vi "rsidr_core_global.vi"() -> ()   [LabVIEW 2020, in "Rohde&Schwarz CMWXP NR FR1 Measurement.lvlib"]
doc: "This Global variable contains driver's:\n- Attributes\n- Range Tables\n- Repeated Capabilities"
uses:
  <instrlib>/Rohde&Schwarz CMWXP NR FR1 Measurement/Rohde&Schwarz CMWXP NR FR1 Measurement.lvlib
panel:
  out "Attributes":T1(array[cluster])=[{"Level"=1, "Class Only"=TRUE, "Identifier"="", "Descriptive Name"="Configuration", "Data Type"=enum."ViInt32", "Command"="", "Access"=enum."Read Only", "Range Table"="", "Read Callback"="", "Write Callback"="", "Range Callback"="", "Check Callback"="", "Rngtable Callback"="", "Coerce Callback"="", "Supported Models"="", "Instrument Options"="", "Check Status Callback"="", "Flags"=0, "Help"="Contains attributes for configuring NR FR 1 Measurement."}, {"Level"=2, "Class Only"=FALSE, "Identifier"="RSCMWXPNRFR1M_ATTR_SIGNAL_PATH", "Descriptive Name"="Signal Path", "Data Type"=enum."RawString", "Command"="ROUT:NRS:MEAS{instance}:SCEN:SAL", "Access"=enum."Read/Write", "Range Table"="", "Read Callback"="", "Write Callback"="", "Range Callback"="", "Check Callback"="", "Rngtable Callback"="", "Coerce Callback"="", "Supported Models"="", "Instrument Options"="", "Check Status Callback"="", "Flags"=0, "Help"="Selects the signal path for the measured signal.\nValue combinations:\nRF 1 COM and RF 2 COM are compatible with TX 1 and TX 3.RF 3 COM and RF 4 COM are compatible with TX 2 and TX 4.\nNote: This command is an interim solution. It is planned to replace this command in a later software version.\n\nSyntax:\nROUTe:NRSub:MEAS<i>:SCENario:SALone <RXConnector>, <RFConverter>\n\n<RXConnector>\nRF connector for the input path\nSingle R&S CMW500: RF<n>C for RF <n> COM\nCMWflexx: R<a><b>C for CMW <a>, connector RF <b> COM\nValid Values:\nRF1C | RF2C | RF3C | RF4C | R11C | R12C | R13C | R14C | R21C | R22C | R23C | R24C | R31C | R32C | R33C | R34C | R41C | R42C | R43C | R44C\n\n<RFConverter>\nRX module for the input path\nSingle R&S CMW500: TX1 to TX4\nCMWflexx: TX<a><b> for CMW <a>, TX <b>\nValid Values:\nTX1 | TX2 | TX3 | TX4 | TX11 | TX12 | TX13 | TX14 | TX21 | TX22 | TX23 | TX24 | TX31 | TX32 | TX33 | TX34 | TX41 | TX42 | TX43 | TX44\n\nAvailable Repeated Capabilities:\ninstance: i0, i1, i2, i3, i4, i5, i6, i7, i8, i9, i10, i11, i12, i13, i14, i15, i16, i17, i18, i19, i20, i21, i22, i23, i24, i25, i26, i27, i28, i29, i30, i31, i32\r\n\nRemote-control command(s):\nROUTe:NRSub:MEAS<i>:SCENario:SALone"}, {"Level"=2, "Class Only"=FALSE, "Identifier"="RSCMWXPNRFR1M_ATTR_CONNECTOR", "Descriptive Name"="Connector", "Data Type"=enum."ViInt32", "Command"="CONF:NRS:MEAS{instance}:SPAT", "Access"=enum."Read/Write", "Range Table"="rsCmwxpNrFr1M_rngConnector", "Read Callback"="", "Write Callback"="", "Range Callback"="", "Check Callback"="", "Rngtable Callback"="", "Coerce Callback"="", "Supported Models"="", "Instrument Options"="", "Check Status Callback"="", "Flags"=0, "Help"="Selects between a standalone measurement and a measurement with coupling to signaling settings (cell settings of the network configuration).\n\nAvailable Repeated Capabilities:\ninstance: i0, i1, i2, i3, i4, i5, i6, i7, i8, i9, i10, i11, i12, i13, i14, i15, i16, i17, i18, i19, i20, i21, i22, i23, i24, i25, i26, i27, i28, i29, i30, i31, i32\r\n\nRemote-control command(s):\nCONFigure:NRSub:MEAS<i>:SPATh"}, {"Level"=2, "Class Only"=FALSE, "Identifier"="RSCMWXPNRFR1M_ATTR_EXTERNAL_ATTENUATION", "Descriptive Name"="External Attenuation", "Data Type"=enum."ViReal64", "Command"="CONF:NRS:MEAS{instance}:RFS:EATT", "Access"=enum."Read/Write", "Range Table"="rsCmwxpNrFr1M_rngExtAtt", "Read Callback"="", "Write Callback"="", "Range Callback"="", "Check Callback"="", "Rngtable Callback"="", "Coerce Callback"="", "Supported Models"="", "Instrument Options"="", "Check Status Callback"="", "Flags"=0, "Help"="Defines an external attenuation (or gain, if the value is negative), to be applied to the input connector.\n\nAvailable Repeated Capabilities:\ninstance: i0, i1, i2, i3, i4, i5, i6, i7, i8, i9, i10, i11, i12, i13, i14, i15, i16, i17, i18, i19, i20, i21, i22, i23, i24, i25, i26, i27, i28, i29, i30, i31, i32\r\n\nRemote-control command(s):\nCONFigure:NRSub:MEAS<i>:RFSettings:EATTenuation"}, {"Level"=2, "Class Only"=FALSE, "Identifier"="RSCMWXPNRFR1M_ATTR_BAND", "Descriptive Name"="Band", "Data Type"=enum."ViInt32", "Command"="CONF:NRS:MEAS{instance}:BAND", "Access"=enum."Read/Write", "Range Table"="rsCmwxpNrFr1M_rngBand", "Read Callback"="rscmwxpnrfr1m_OperatingBand_ReadCallback.vi", "Write Callback"="rscmwxpnrfr1m_OperatingBand_WriteCallback.vi", "Range Callback"="", "Check Callback"="", "Rngtable Callback"="", "Coerce Callback"="", "Supported Models"="", "Instrument Options"="", "Check Status Callback"="", "Flags"=0, "Help"="Selects the operating band (OB). The allowed input range depends on the duplex mode (FDD or TDD).\n\nAvailable Repeated Capabilities:\ninstance: i0, i1, i2, i3, i4, i5, i6, i7, i8, i9, i10, i11, i12, i13, i14, i15, i16, i17, i18, i19, i20, i21, i22, i23, i24, i25, i26, i27, i28, i29, i30, i31, i32\r\n\nRemote-control command(s):\nCONFigure:NRSub:MEAS<i>:BAND"}, {"Level"=2, "Class Only"=FALSE, "Identifier"="RSCMWXPNRFR1M_ATTR_FREQUENCY", "Descriptive Name"="Frequency", "Data Type"=enum."ViReal64", "Command"="CONF:NRS:MEAS{instance}:RFS:FREQ", "Access"=enum."Read/Write", "Range Table"="", "Read Callback"="", "Write Callback"="", "Range Callback"="", "Check Callback"="", "Rngtable Callback"="", "Coerce Callback"="", "Supported Models"="", "Instrument Options"="", "Check Status Callback"="", "Flags"=0, "Help"="Selects the center frequency of the measured carrier.\n\nAvailable Repeated Capabilities:\ninstance: i0, i1, i2, i3, i4, i5, i6, i7, i8, i9, i10, i11, i12, i13, i14, i15, i16, i17, i18, i19, i20, i21, i22, i23, i24, i25, i26, i27, i28, i29, i30, i31, i32\r\n\nRemote-control command(s):\nCONFigure:NRSub:MEAS<i>:RFSettings:FREQuency"}, {"Level"=2, "Class Only"=FALSE, "Identifier"="RSCMWXPNRFR1M_ATTR_FREQUENCY_OFFSET", "Descriptive Name"="Frequency Offset", "Data Type"=enum."ViReal64", "Command"="CONF:NRS:MEAS{instance}:RFS:FOFF", "Access"=enum."Read/Write", "Range Table"="rsCmwxpNrFr1M_rngFrequencyOffset", "Read Callback"="", "Write Callback"="", "Range Callback"="", "Check Callback"="", "Rngtable Callback"="", "Coerce Callback"="", "Supported Models"="", "Instrument Options"="", "Check Status Callback"="", "Flags"=0, "Help"="Specifies a positive or negative frequency offset to be added to the carrier center frequency.\n\nAvailable Repeated Capabilities:\ninstance: i0, i1, i2, i3, i4, i5, i6, i7, i8, i9, i10, i11, i12, i13, i14, i15, i16, i17, i18, i19, i20, i21, i22, i23, i24, i25, i26, i27, i28, i29, i30, i31, i32\r\n\nRemote-control command(s):\nCONFigure:NRSub:MEAS<i>:RFSettings:FOFFset"}, {"Level"=2, "Class Only"=FALSE, "Identifier"="RSCMWXPNRFR1M_ATTR_EXPECTED_NOMINAL_POWER", "Descriptive Name"="Expected Nominal Power", "Data Type"=enum."ViReal64", "Command"="CONF:NRS:MEAS{instance}:RFS:ENP", "Access"=enum."Read/Write", "Range Table"="", "Read Callback"="", "Write Callback"="", "Range Callback"="", "Check Callback"="", "Rngtable Callback"="", "Coerce Callback"="", "Supported Models"="", "Instrument Options"="", "Check Status Callback"="", "Flags"=0, "Help"="Sets the expected nominal power of the measured RF signal.\n\nAvailable Repeated Capabilities:\ninstance: i0, i1, i2, i3, i4, i5, i6, i7, i8, i9, i10, i11, i12, i13, i14, i15, i16, i17, i18, i19, i20, i21, i22, i23, i24, i25, i26, i27, i28, i29, i30, i31, i32\r\n\nRemote-control command(s):\nCONFigure:NRSub:MEAS<i>:RFSettings:ENPower"}, {"Level"=2, "Class Only"=FALSE, "Identifier"="RSCMWXPNRFR1M_ATTR_USER_MARGIN", "Descriptive Name"="User Margin", "Data Type"=enum."ViReal64", "Command"="CONF:NRS:MEAS{instance}:RFS:UMAR", "Access"=enum."Read/Write", "Range Table"="", "Read Callback"="", "Write Callback"="", "Range Callback"="", "Check Callback"="", "Rngtable Callback"="", "Coerce Callback"="", "Supported Models"="", "Instrument Options"="", "Check Status Callback"="", "Flags"=0, "Help"="Sets the margin that the measurement adds to the expected nominal power to determine the reference power. The reference power minus the external input attenuation must be within the power range of the selected input connector. Refer to the data sheet.\n\nAvailable Repeated Capabilities:\ninstance: i0, i1, i2, i3, i4, i5, i6, i7, i8, i9, i10, i11, i12, i13, i14, i15, i16, i17, i18, i19, i20, i21, i22, i23, i24, i25, i26, i27, i28, i29, i30, i31, i32\r\n\nRemote-control command(s):\nCONFigure:NRSub:MEAS<i>:RFSettings:UMARgin"}, {"Level"=2, "Class Only"=FALSE, "Identifier"="RSCMWXPNRFR1M_ATTR_MIXER_LEVEL_OFFSET", "Descriptive Name"="Mixer Level Offset", "Data Type"=enum."ViReal64", "Command"="CONF:NRS:MEAS{instance}:RFS:MLOF", "Access"=enum."Read/Write", "Range Table"="rsCmwxpNrFr1M_rngMixerLevelOffset", "Read Callback"="", "Write Callback"="", "Range Callback"="", "Check Callback"="", "Rngtable Callback"="", "Coerce Callback"="", "Supported Models"="", "Instrument Options"="", "Check Status Callback"="", "Flags"=0, "Help"="Varies the input level of the mixer in the analyzer path.\n\nAvailable Repeated Capabilities:\ninstance: i0, i1, i2, i3, i4, i5, i6, i7, i8, i9, i10, i11, i12, i13, i14, i15, i16, i17, i18, i19, i20, i21, i22, i23, i24, i25, i26, i27, i28, i29, i30, i31, i32\r\n\nRemote-control command(s):\nCONFigure:NRSub:MEAS<i>:RFSettings:MLOFfset"}, {"Level"=2, "Class Only"=FALSE, "Identifier"="RSCMWXPNRFR1M_ATTR_RF_UPCONVERSION", "Descriptive Name"="RF Upconversion", "Data Type"=enum."RawString", "Command"="CONF:NRS:MEAS{instance}:MEV:PCOM", "Access"=enum."Read/Write", "Range Table"="", "Read Callback"="", "Write Callback"="", "Range Callback"="", "Check Callback"="", "Rngtable Callback"="", "Coerce Callback"="", "Supported Models"="", "Instrument Options"="", "Check Status Callback"="", "Flags"=0, "Help"="Specifies the phase compensation applied by the UE during the modulation and upconversion.\n\nSyntax:\nCONFigure:NRSub:MEAS<i>:MEValuation:PCOMp <PhaseComp>, <UserDefFreq>\n\n<PhaseComp>\nValid Values:\nOFF: no phase compensation\nCAF: phase compensation for carrier frequency\nUDEF: phase compensation for frequency <UserDefFreq>\n \n<UserDefFreq>\n numeric\nFrequency for <PhaseComp> = UDEF\nValid Values: 0 Hz to 10E+9 Hz\n\nAvailable Repeated Capabilities:\ninstance: i0, i1, i2, i3, i4, i5, i6, i7, i8, i9, i10, i11, i12, i13, i14, i15, i16, i17, i18, i19, i20, i21, i22, i23, i24, i25, i26, i27, i28, i29, i30, i31, i32\r\n\nRemote-control command(s):\nCONFigure:NRSub:MEAS<i>:MEValuation:PCOMp"}, {"Level"=2, "Class Only"=FALSE, "Identifier"="RSCMWXPNRFR1M_ATTR_DUPLEX_MODE", "Descriptive Name"="Duplex Mode", "Data Type"=enum."ViInt32", "Command"="CONF:NRS:MEAS{instance}:MEV:DMOD", "Access"=enum."Read/Write", "Range Table"="rsCmwxpNrFr1M_rngDuplexMode", "Read Callback"="", "Write Callback"="", "Range Callback"="", "Check Callback"="", "Rngtable Callback"="", "Coerce Callback"="", "Supported Models"="", "Instrument Options"="", "Check Status Callback"="", "Flags"=0, "Help"="Selects the duplex mode of the signal: FDD or TDD.\n\nAvailable Repeated Capabilities:\ninstance: i0, i1, i2, i3, i4, i5, i6, i7, i8, i9, i10, i11, i12, i13, i14, i15, i16, i17, i18, i19, i20, i21, i22, i23, i24, i25, i26, i27, i28, i29, i30, i31, i32\r\n\nRemote-control command(s):\nCONFigure:NRSub:MEAS<i>:MEValuation:DMODe"}, {"Level"=2, "Class Only"=FALSE, "Identifier"="RSCMWXPNRFR1M_ATTR_EN_DC_MODE", "Descriptive Name"="EN-DC Mode", "Data Type"=enum."ViBoolean", "Command"="CONF:NRS:MEAS{instance}:MEV:ENDC", "Access"=enum."Read/Write", "Range Table"="", "Read Callback"="", "Write Callback"="", "Range Callback"="", "Check Callback"="", "Rngtable Callback"="", "Coerce Callback"="", "Supported Models"="", "Instrument Options"="", "Check Status Callback"="", "Flags"=0, "Help"="Enables or disables the EN-DC mode of the measurement.\n\nAvailable Repeated Capabilities:\ninstance: i0, i1, i2, i3, i4, i5, i6, i7, i8, i9, i10, i11, i12, i13, i14, i15, i16, i17, i18, i19, i20, i21, i22, i23, i24, i25, i26, i27, i28, i29, i30, i31, i32\r\n\nRemote-control command(s):\nCONFigure:NRSub:MEAS<i>:MEValuation:ENDC"}, {"Level"=2, "Class Only"=FALSE, "Identifier"="RSCMWXPNRFR1M_ATTR_EN_DC_LTE", "Descriptive Name"="EN-DC LTE", "Data Type"=enum."RawString", "Command"="CONF:NRS:MEAS{instance}:MEV:ENDC:EUTR", "Access"=enum."Read/Write", "Range Table"="", "Read Callback"="", "Write Callback"="", "Range Callback"="", "Check Callback"="", "Rngtable Callback"="", "Coerce Callback"="", "Supported Models"="", "Instrument Options"="", "Check Status Callback"="", "Flags"=0, "Help"="Configures LTE settings for EN-DC.\n\nSyntax:\nCONFigure:NRSub:MEAS<i>:MEValuation:ENDC:EUTRa <ChannelBW>, <CarrierPosition>\n\n<ChannelBW>\nChannel bandwidth in MHz (5 MHz to 20 MHz)\nValid Values:\nB005 | B010 | B015 | B020\n\n<CarrierPosition>\nPosition of LTE carrier left (LONR) or right (RONR) of NR carrier.\nValid Values:\nLONR | RONR\n\nAvailable Repeated Capabilities:\ninstance: i0, i1, i2, i3, i4, i5, i6, i7, i8, i9, i10, i11, i12, i13, i14, i15, i16, i17, i18, i19, i20, i21, i22, i23, i24, i25, i26, i27, i28, i29, i30, i31, i32\r\n\nRemote-control command(s):\nCONFigure:NRSub:MEAS<i>:MEValuation:ENDC:EUTRa"}, {"Level"=2, "Class Only"=FALSE, "Identifier"="RSCMWXPNRFR1M_ATTR_TX_BANDWIDTH_OFFSET", "Descriptive Name"="Tx Bandwidth Offset", "Data Type"=enum."ViInt32", "Command"="CONF:NRS:MEAS{instance}:CC{CC}:TXBW:OFFS", "Access"=enum."Read/Write", "Range Table"="rsCmwxpNrFr1M_rngTxBWOffset", "Read Callback"="", "Write Callback"="", "Range Callback"="", "Check Callback"="", "Rngtable Callback"="", "Coerce Callback"="", "Supported Models"="", "Instrument Options"="", "Check Status Callback"="", "Flags"=0, "Help"="Specifies the offset to carrier (TxBW offset) of carrier <no>.\n\nAvailable Repeated Capabilities:\ninstance: i0, i1, i2, i3, i4, i5, i6, i7, i8, i9, i10, i11, i12, i13, i14, i15, i16, i17, i18, i19, i20, i21, i22, i23, i24, i25, i26, i27, i28, i29, i30, i31, i32\r\nCC: cc1, cc2\r\n\nRemote-control command(s):\nCONFigure:NRSub:MEAS<i>[:CC<no>]:TXBWidth:OFFSet"}, {"Level"=2, "Class Only"=TRUE, "Identifier"="", "Descriptive Name"="Signal Settings", "Data Type"=enum."ViInt32", "Command"="", "Access"=enum."Read Only", "Range Table"="", "Read Callback"="", "Write Callback"="", "Range Callback"="", "Check Callback"="", "Rngtable Callback"="", "Coerce Callback"="", "Supported Models"="", "Instrument Options"="", "Check Status Callback"="", "Flags"=0, "Help"="Describe properties of the measured NR signal, that are needed for synchronization and decoding."}, {"Level"=3, "Class Only"=TRUE, "Identifier"="", "Descriptive Name"="TDD UL-DL Configuration", "Data Type"=enum."ViInt32", "Command"="", "Access"=enum."Read Only", "Range Table"="", "Read Callback"="", "Write Callback"="", "Range Callback"="", "Check Callback"="", "Rngtable Callback"="", "Coerce Callback"="", "Supported Models"="", "Instrument Options"="", "Check Status Callback"="", "Flags"=0, "Help"="Settings that configure the UL-DL pattern."}, {"Level"=4, "Class Only"=FALSE, "Identifier"="RSCMWXPNRFR1M_ATTR_UL_DL_PERIODICITY", "Descriptive Name"="UL-DL Periodicity", "Data Type"=enum."ViInt32", "Command"="CONF:NRS:MEAS{instance}:ULDL:PER", "Access"=enum."Read/Write", "Range Table"="rsCmwxpNrFr1M_rngPeriodicity", "Read Callback"="", "Write Callback"="", "Range Callback"="", "Check Callback"="", "Rngtable Callback"="", "Coerce Callback"="", "Supported Models"="", "Instrument Options"="", "Check Status Callback"="", "Flags"=0, "Help"="Configures the periodicity of the TDD UL-DL pattern.\n\nAvailable Repeated Capabilities:\ninstance: i0, i1, i2, i3, i4, i5, i6, i7, i8, i9, i10, i11, i12, i13, i14, i15, i16, i17, i18, i19, i20, i21, i22, i23, i24, i25, i26, i27, i28, i29, i30, i31, i32\r\n\nRemote-control command(s):\nCONFigure:NRSub:MEAS<i>:ULDL:PERiodicity"}, {"Level"=4, "Class Only"=FALSE, "Identifier"="RSCMWXPNRFR1M_ATTR_UL_DL_PATTERN", "Descriptive Name"="UL-DL Pattern", "Data Type"=enum."RawString", "Command"="CONF:NRS:MEAS{instance}:ULDL:PATT", "Access"=enum."Write Only", "Range Table"="", "Read Callback"="", "Write Callback"="", "Range Callback"="", "Check Callback"="", "Rngtable Callback"="", "Coerce Callback"="", "Supported Models"="", "Instrument Options"="", "Check Status Callback"="", "Flags"=0, "Help"="Configures the UL-DL pattern for the <SCSpacing>.\n\nSyntax:\nCONFigure:NRMMw:MEAS<i>:ULDL:PATTern <SCSpacing>, <DLSlots>, <DLSymbols>, <ULSlots>, <ULSymbols>\n\n<SCSpacing>\nSubcarrier spacing for which the other settings apply.\nValid Values:\nS60K\nS120k\n\n<DLSlots>\nnumeric\nSpecifies nrofDownlinkSlots.\nValid Values:  0  to  78 \n\n<DLSymbols>\n numeric\nSpecifies nrofDownlinkSymbols.\nValid Values: 0 to 14 \n\n<ULSlots>\n numeric\nSpecifies nrofUplinkSlots.\nValid Values: 1 to 80 \n\n<ULSymbols>\nnumeric\nSpecifies nrofUplinkSymbols.\nValid Values: 0 to 14\n\nAvailable Repeated Capabilities:\ninstance: i0, i1, i2, i3, i4, i5, i6, i7, i8, i9, i10, i11, i12, i13, i14, i15, i16, i17, i18, i19, i20, i21, i22, i23, i24, i25, i26, i27, i28, i29, i30, i31, i32\r\n\nRemote-control command(s):\nCONFigure:NRSub:MEAS<i>:ULDL:PATTern"}, {"Level"=4, "Class Only"=FALSE, "Identifier"="RSCMWXPNRFR1M_ATTR_HIDDEN_QUERY_UL_DL_PATTERN", "Descriptive Name"="Query UL-DL Pattern", "Data Type"=enum."RawString", "Command"="CONF:NRS:MEAS{instance}:ULDL:PATT?", "Access"=enum."Read Only", "Range Table"="", "Read Callback"="", "Write Callback"="", "Range Callback"="", "Check Callback"="", "Rngtable Callback"="", "Coerce Callback"="", "Supported Models"="", "Instrument Options"="", "Check Status Callback"="", "Flags"=8, "Help"="Retrives the UL-DL pattern for the <SCSpacing>.\n\nSyntax:\nCONFigure:NRMMw:MEAS<i>:ULDL:PATTern? <SCSpacing>\n\nParameters:\n<SCSpacing>\nSubcarrier spacing for which the other settings apply.\nValid Values:\nS60K\nS120k\n\nResponse:\n<DLSlots>\nnumeric\nSpecifies nrofDownlinkSlots.\nValid Values:  0  to  78 \n\n<DLSymbols>\n numeric\nSpecifies nrofDownlinkSymbols.\nValid Values: 0 to 14 \n\n<ULSlots>\n numeric\nSpecifies nrofUplinkSlots.\nValid Values: 1 to 80 \n\n<ULSymbols>\nnumeric\nSpecifies nrofUplinkSymbols.\nValid Values: 0 to 14\n\nAvailable Repeated Capabilities:\ninstance: i0, i1, i2, i3, i4, i5, i6, i7, i8, i9, i10, i11, i12, i13, i14, i15, i16, i17, i18, i19, i20, i21, i22, i23, i24, i25, i26, i27, i28, i29, i30, i31, i32\r\n\nRemote-control command(s):\nCONFigure:NRSub:MEAS<i>:ULDL:PATTern?"}, {"Level"=3, "Class Only"=TRUE, "Identifier"="", "Descriptive Name"="General Carrier Settings", "Data Type"=enum."ViInt32", "Command"="", "Access"=enum."Read Only", "Range Table"="", "Read Callback"="", "Write Callback"="", "Range Callback"="", "Check Callback"="", "Rngtable Callback"="", "Coerce Callback"="", "Supported Models"="", "Instrument Options"="", "Check Status Callback"="", "Flags"=0, "Help"="General carrier settings."}, {"Level"=4, "Class Only"=FALSE, "Identifier"="RSCMWXPNRFR1M_ATTR_CHANNEL_BANDWIDTH", "Descriptive Name"="Channel Bandwidth", "Data Type"=enum."ViInt32", "Command"="CONF:NRS:MEAS{instance}:CC{CC}:CBAN", "Access"=enum."Read/Write", "Range Table"="rsCmwxpNrFr1M_rngChannelBandwidth", "Read Callback"="", "Write Callback"="", "Range Callback"="", "Check Callback"="", "Rngtable Callback"="", "Coerce Callback"="", "Supported Models"="", "Instrument Options"="", "Check Status Callback"="", "Flags"=0, "Help"="Specifies the channel bandwidth of carrier <no>.\n\nAvailable Repeated Capabilities:\ninstance: i0, i1, i2, i3, i4, i5, i6, i7, i8, i9, i10, i11, i12, i13, i14, i15, i16, i17, i18, i19, i20, i21, i22, i23, i24, i25, i26, i27, i28, i29, i30, i31, i32\r\nCC: cc1, cc2\r\n\nRemote-control command(s):\nCONFigure:NRSub:MEAS<i>[:CC<no>]:CBANdwidth"}, {"Level"=4, "Class Only"=FALSE, "Identifier"="RSCMWXPNRFR1M_ATTR_PHYSICAL_CELL_ID", "Descriptive Name"="Physical Cell ID", "Data Type"=enum."ViInt32", "Command"="CONF:NRS:MEAS{instance}:CC{CC}:PLC", "Access"=enum."Read/Write", "Range Table"="rsCmwxpNrFr1M_rngPhysicalCellID", "Read Callback"="", "Write Callback"="", "Range Callback"="", "Check Callback"="", "Rngtable Callback"="", "Coerce Callback"="", "Supported Models"="", "Instrument Options"="", "Check Status Callback"="", "Flags"=0, "Help"="Specifies the physical cell ID of carrier <no>.\n\nAvailable Repeated Capabilities:\ninstance: i0, i1, i2, i3, i4, i5, i6, i7, i8, i9, i10, i11, i12, i13, i14, i15, i16, i17, i18, i19, i20, i21, i22, i23, i24, i25, i26, i27, i28, i29, i30, i31, i32\r\nCC: cc1, cc2\r\n\nRemote-control command(s):\nCONFigure:NRSub:MEAS<i>[:CC<no>]:PLCid"}, {"Level"=4, "Class Only"=FALSE, "Identifier"="RSCMWXPNRFR1M_ATTR_DMRS_TYPE_A_POSITION", "Descriptive Name"="DMRS Type A Position", "Data Type"=enum."ViInt32", "Command"="CONF:NRS:MEAS{instance}:CC{CC}:TAP", "Access"=enum."Read/Write", "Range Table"="rsCmwxpNrFr1M_rngTypeAPosition", "Read Callback"="", "Write Callback"="", "Range Callback"="", "Check Callback"="", "Rngtable Callback"="", "Coerce Callback"="", "Supported Models"="", "Instrument Options"="", "Check Status Callback"="", "Flags"=0, "Help"="Specifies the 'dmrs-TypeA-Position' for carrier <no>.\n\nAvailable Repeated Capabilities:\ninstance: i0, i1, i2, i3, i4, i5, i6, i7, i8, i9, i10, i11, i12, i13, i14, i15, i16, i17, i18, i19, i20, i21, i22, i23, i24, i25, i26, i27, i28, i29, i30, i31, i32\r\nCC: cc1, cc2\r\n\nRemote-control command(s):\nCONFigure:NRSub:MEAS<i>[:CC<no>]:TAPosition"}, {"Level"=4, "Class Only"=FALSE, "Identifier"="RSCMWXPNRFR1M_ATTR_SUBCARRIER_SPACING", "Descriptive Name"="Subcarrier Spacing", "Data Type"=enum."ViInt32", "Command"="CONF:NRS:MEAS{instance}:CCAL:TXBW:SCSP", "Access"=enum."Read/Write", "Range Table"="rsCmwxpNrFr1M_rngSubcarrierSpacing", "Read Callback"="", "Write Callback"="", "Range Callback"="", "Check Callback"="", "Rngtable Callback"="", "Coerce Callback"="", "Supported Models"="", "Instrument Options"="", "Check Status Callback"="", "Flags"=0, "Help"="Selects the subcarrier spacing for the measurement, for all carriers.\n\nAvailable Repeated Capabilities:\ninstance: i0, i1, i2, i3, i4, i5, i6, i7, i8, i9, i10, i11, i12, i13, i14, i15, i16, i17, i18, i19, i20, i21, i22, i23, i24, i25, i26, i27, i28, i29, i30, i31, i32\r\n\nRemote-control command(s):\nCONFigure:NRSub:MEAS<i>:CCALl:TXBWidth:SCSPacing"}, {"Level"=3, "Class Only"=TRUE, "Identifier"="", "Descriptive Name"="Bandwidth Parts", "Data Type"=enum."ViInt32", "Command"="", "Access"=enum."Read Only", "Range Table"="", "Read Callback"="", "Write Callback"="", "Range Callback"="", "Check Callback"="", "Rngtable Callback"="", "Coerce Callback"="", "Supported Models"="", "Instrument Options"="", "Check Status Callback"="", "Flags"=0, "Help"="Contains attributes for Bandwidth Parts."}, {"Level"=4, "Class Only"=FALSE, "Identifier"="RSCMWXPNRFR1M_ATTR_BANDWIDTH_PART", "Descriptive Name"="Bandwidth Part", "Data Type"=enum."RawString", "Command"="CONF:NRS:MEAS{instance}:CC{CC}:BWP", "Access"=enum."Write Only", "Range Table"="", "Read Callback"="", "Write Callback"="", "Range Callback"="", "Check Callback"="", "Rngtable Callback"="", "Coerce Callback"="", "Supported Models"="", "Instrument Options"="", "Check Status Callback"="", "Flags"=0, "Help"="Configures basic properties of the <BWP> on carrier <CC>.\n\nSyntax:\nCONFigure:NRSub:MEAS<i>[:CC<no>]:BWPart <BWP>, <SCSpacing>, <CyclicPrefix>, <NumberRB>, <StartRB>\n\n<BWP>\nSelects BWP.\nValid Values:\nBWP0\n\n<SCSpacing>\nSubcarrier spacing 15 kHz, 30 kHz, 60 kHz.\nValid Values:\nS15K\nS30K\nS60K\n\n<CyclicPrefix>\nOnly normal CP is supported.\nValid Values:\nNORM\nEXT\n\n<NumberRB>\nNumber of RBs in the bandwidth part.\ninteger\nValid Values: 11 to 273 \n\n<StartRB>\nIndex of the first RB in the bandwidth part.\ninteger\nValid Values: 0 to 262\n\nAvailable Repeated Capabilities:\ninstance: i0, i1, i2, i3, i4, i5, i6, i7, i8, i9, i10, i11, i12, i13, i14, i15, i16, i17, i18, i19, i20, i21, i22, i23, i24, i25, i26, i27, i28, i29, i30, i31, i32\r\nCC: cc1, cc2\r\n\nRemote-control command(s):\nCONFigure:NRSub:MEAS<i>[:CC<no>]:BWPart"}, {"Level"=4, "Class Only"=FALSE, "Identifier"="RSCMWXPNRFR1M_ATTR_HIDDEN_QUERY_BANDWIDTH_PART", "Descriptive Name"="Query Bandwidth Part", "Data Type"=enum."RawString", "Command"="CONF:NRS:MEAS{instance}:CC{CC}:BWP?", "Access"=enum."Read Only", "Range Table"="", "Read Callback"="", "Write Callback"="", "Range Callback"="", "Check Callback"="", "Rngtable Callback"="", "Coerce Callback"="", "Supported Models"="", "Instrument Options"="", "Check Status Callback"="", "Flags"=8, "Help"="Queries basic properties of the <BWP> on carrier <CC>.\n\nSyntax:\nCONFigure:NRSub:MEAS<i>[:CC<no>]:BWPart? <BWP>\n\nParameters:\n<BWP>\nSelects BWP.\nValid Values:\nBWP0\n\nResponse:\n<SCSpacing>\nSubcarrier spacing 15 kHz, 30 kHz, 60 kHz.\nValid Values:\nS15K\nS30K\nS60K\n\n<CyclicPrefix>\nOnly normal CP is supported.\nValid Values:\nNORM\nEXT\n\n<NumberRB>\nNumber of RBs in the bandwidth part.\ninteger\nValid Values: 11 to 273 \n\n<StartRB>\nIndex of the first RB in the bandwidth part.\ninteger\nValid Values: 0 to 262\n\nAvailable Repeated Capabilities:\ninstance: i0, i1, i2, i3, i4, i5, i6, i7, i8, i9, i10, i11, i12, i13, i14, i15, i16, i17, i18, i19, i20, i21, i22, i23, i24, i25, i26, i27, i28, i29, i30, i31, i32\r\nCC: cc1, cc2\r\n\nRemote-control command(s):\nCONFigure:NRSub:MEAS<i>[:CC<no>]:BWPart?"}, {"Level"=4, "Class Only"=FALSE, "Identifier"="RSCMWXPNRFR1M_ATTR_DMRS_FOR_MAPPING_TYPE_A", "Descriptive Name"="DMRS For Mapping Type A", "Data Type"=enum."RawString", "Command"="CONF:NRS:MEAS{instance}:CC{CC}:BWP:PUSC:DMTA", "Access"=enum."Write Only", "Range Table"="", "Read Callback"="", "Write Callback"="", "Range Callback"="", "Check Callback"="", "Rngtable Callback"="", "Coerce Callback"="", "Supported Models"="", "Instrument Options"="", "Check Status Callback"="", "Flags"=0, "Help"="Configures the DM-RS for mapping type A. The settings apply to the <BWP> on carrier <no>.\n\nSyntax:\nCONFigure:NRSub:MEAS<i>[:CC<no>]:BWPart:PUSCh:DMTA <BWP>, <ConfigType>, <AddPosition>, <MaxLength>\n\n<BWP>\nSelects BWP.\nValid Values:\nBWP0\n\n<ConfigType>\nDM-RS setting 'dmrs-Type'.\nnumeric\nValid Values: 1 to 2 \n \n<AddPosition>\nDM-RS setting 'dmrs-AdditionalPosition'.\nnumeric\nValid Values: 0 to 3\n\n<MaxLength>\nDM-RS setting 'maxLength'.\nnumeric\nValid Values: 1\n\nAvailable Repeated Capabilities:\ninstance: i0, i1, i2, i3, i4, i5, i6, i7, i8, i9, i10, i11, i12, i13, i14, i15, i16, i17, i18, i19, i20, i21, i22, i23, i24, i25, i26, i27, i28, i29, i30, i31, i32\r\nCC: cc1, cc2\r\n\nRemote-control command(s):\nCONFigure:NRSub:MEAS<i>[:CC<no>]:BWPart:PUSCh:DMTA"}, {"Level"=4, "Class Only"=FALSE, "Identifier"="RSCMWXPNRFR1M_ATTR_HIDDEN_QUERY_DMRS_FOR_MAPPING_TYPE_A", "Descriptive Name"="Query DMRS For Mapping Type A", "Data Type"=enum."RawString", "Command"="CONF:NRS:MEAS{instance}:CC{CC}:BWP:PUSC:DMTA?", "Access"=enum."Read Only", "Range Table"="", "Read Callback"="", "Write Callback"="", "Range Callback"="", "Check Callback"="", "Rngtable Callback"="", "Coerce Callback"="", "Supported Models"="", "Instrument Options"="", "Check Status Callback"="", "Flags"=8, "Help"="Queries the DM-RS for mapping type A. The settings apply to the <BWP> on carrier <no>.\n\nSyntax:\nCONFigure:NRSub:MEAS<i>[:CC<no>]:BWPart:PUSCh:DMTA? <BWP>\n\nParameters:\n<BWP>\nSelects BWP.\nValid Values:\nBWP0\n\nResponse:\n<ConfigType>\nDM-RS setting 'dmrs-Type'.\nnumeric\nValid Values: 1 to 2 \n \n<AddPosition>\nDM-RS setting 'dmrs-AdditionalPosition'.\nnumeric\nValid Values: 0 to 3\n\n<MaxLength>\nDM-RS setting 'maxLength'.\nnumeric\nValid Values: 1\n\nAvailable Repeated Capabilities:\ninstance: i0, i1, i2, i3, i4, i5, i6, i7, i8, i9, i10, i11, i12, i13, i14, i15, i16, i17, i18, i19, i20, i21, i22, i23, i24, i25, i26, i27, i28, i29, i30, i31, i32\r\nCC: cc1, cc2\r\n\nRemote-control command(s):\nCONFigure:NRSub:MEAS<i>[:CC<no>]:BWPart:PUSCh:DMTA?"}, {"Level"=4, "Class Only"=FALSE, "Identifier"="RSCMWXPNRFR1M_ATTR_DMRS_FOR_MAPPING_TYPE_B", "Descriptive Name"="DMRS For Mapping Type B", "Data Type"=enum."RawString", "Command"="CONF:NRS:MEAS{instance}:CC{CC}:BWP:PUSC:DMTB", "Access"=enum."Write Only", "Range Table"="", "Read Callback"="", "Write Callback"="", "Range Callback"="", "Check Callback"="", "Rngtable Callback"="", "Coerce Callback"="", "Supported Models"="", "Instrument Options"="", "Check Status Callback"="", "Flags"=0, "Help"="Configures the DM-RS for mapping type B. The settings apply to the <BWP> on carrier <no>.\n\nSyntax:\nCONFigure:NRMMw:MEAS<i>[:CC<no>]:BWPart:PUSCh:DMTA <BWP>, <ConfigType>, <AddPosition>, <MaxLength>\n\n<BWP>\nSelects BWP.\nValid Values:\nBWP0\n\n<ConfigType>\nDM-RS setting 'dmrs-Type'.\nnumeric\nValid Values: 1 to 2 \n \n<AddPosition>\nDM-RS setting 'dmrs-AdditionalPosition'.\nnumeric\nValid Values: 0 to 3\n\n<MaxLength>\nDM-RS setting 'maxLength'.\nnumeric\nValid Values: 1\n\nAvailable Repeated Capabilities:\ninstance: i0, i1, i2, i3, i4, i5, i6, i7, i8, i9, i10, i11, i12, i13, i14, i15, i16, i17, i18, i19, i20, i21, i22, i23, i24, i25, i26, i27, i28, i29, i30, i31, i32\r\nCC: cc1, cc2\r\n\nRemote-control command(s):\nCONFigure:NRSub:MEAS<i>[:CC<no>]:BWPart:PUSCh:DMTB"}, {"Level"=4, "Class Only"=FALSE, "Identifier"="RSCMWXPNRFR1M_ATTR_HIDDEN_QUERY_DMRS_FOR_MAPPING_TYPE_B", "Descriptive Name"="Query DMRS For Mapping Type B", "Data Type"=enum."RawString", "Command"="CONF:NRS:MEAS{instance}:CC{CC}:BWP:PUSC:DMTB?", "Access"=enum."Read Only", "Range Table"="", "Read Callback"="", "Write Callback"="", "Range Callback"="", "Check Callback"="", "Rngtable Callback"="", "Coerce Callback"="", "Supported Models"="", "Instrument Options"="", "Check Status Callback"="", "Flags"=8, "Help"="Queries the DM-RS for mapping type B. The settings apply to the <BWP> on carrier <no>.\n\nSyntax:\nCONFigure:NRSub:MEAS<i>[:CC<no>]:BWPart:PUSCh:DMTB? <BWP>\n\nParameters:\n<BWP>\nSelects BWP.\nValid Values:\nBWP0\n\nResponse:\n<ConfigType>\nDM-RS setting 'dmrs-Type'.\nnumeric\nValid Values: 1 to 2 \n \n<AddPosition>\nDM-RS setting 'dmrs-AdditionalPosition'.\nnumeric\nValid Values: 0 to 3\n\n<MaxLength>\nDM-RS setting 'maxLength'.\nnumeric\nValid Values: 1\n\nAvailable Repeated Capabilities:\ninstance: i0, i1, i2, i3, i4, i5, i6, i7, i8, i9, i10, i11, i12, i13, i14, i15, i16, i17, i18, i19, i20, i21, i22, i23, i24, i25, i26, i27, i28, i29, i30, i31, i32\r\nCC: cc1, cc2\r\n\nRemote-control command(s):\nCONFigure:NRSub:MEAS<i>[:CC<no>]:BWPart:PUSCh:DMTB?"}, {"Level"=4, "Class Only"=FALSE, "Identifier"="RSCMWXPNRFR1M_ATTR_TRANSFORM_PRECODING", "Descriptive Name"="Transform Precoding", "Data Type"=enum."RawString", "Command"="CONF:NRS:MEAS{instance}:CC{CC}:BWP:PUSC:DFTP", "Access"=enum."Write Only", "Range Table"="", "Read Callback"="", "Write Callback"="", "Range Callback"="", "Check Callback"="", "Rngtable Callback"="", "Coerce Callback"="", "Supported Models"="", "Instrument Options"="", "Check Status Callback"="", "Flags"=0, "Help"="Specifies whether the <BWP> on carrier <no> uses a transform precoding function.\n\nSyntax:\n<BWP>\nSelects BWP.\nValid Values:\nBWP0\n\n<Enable>\nValid Values:\nOFF - No transform precoding\nON - With transform precoding\n\nAvailable Repeated Capabilities:\ninstance: i0, i1, i2, i3, i4, i5, i6, i7, i8, i9, i10, i11, i12, i13, i14, i15, i16, i17, i18, i19, i20, i21, i22, i23, i24, i25, i26, i27, i28, i29, i30, i31, i32\r\nCC: cc1, cc2\r\n\nRemote-control command(s):\nCONFigure:NRSub:MEAS<i>[:CC<no>]:BWPart:PUSCh:DFTPrecoding"}, {"Level"=4, "Class Only"=FALSE, "Identifier"="RSCMWXPNRFR1M_ATTR_HIDDEN_QUERY_TRANSFORM_PRECODING", "Descriptive Name"="Query Transform Precoding", "Data Type"=enum."ViBoolean", "Command"="CONF:NRS:MEAS{instance}:CC{CC}:BWP:PUSC:DFTP?", "Access"=enum."Read Only", "Range Table"="", "Read Callback"="", "Write Callback"="", "Range Callback"="", "Check Callback"="", "Rngtable Callback"="", "Coerce Callback"="", "Supported Models"="", "Instrument Options"="", "Check Status Callback"="", "Flags"=8, "Help"="Query whether the <BWP> on carrier <no> uses a transform precoding function.\n\nSyntax:\nCONFigure:NRSub:MEAS<i>[:CC<no>]:BWPart:PUSCh:DFTPrecoding? <BWP>\n\nParameters:\n<BWP>\nSelects bandwidth part.\nValid Values:\nBWP0\n\nAvailable Repeated Capabilities:\ninstance: i0, i1, i2, i3, i4, i5, i6, i7, i8, i9, i10, i11, i12, i13, i14, i15, i16, i17, i18, i19, i20, i21, i22, i23, i24, i25, i26, i27, i28, i29, i30, i31, i32\r\nCC: cc1, cc2\r\n\nRemote-control command(s):\nCONFigure:NRSub:MEAS<i>[:CC<no>]:BWPart:PUSCh:DFTPrecoding?"}, {"Level"=3, "Class Only"=TRUE, "Identifier"="", "Descriptive Name"="Scheduled Slot Allocation", "Data Type"=enum."ViInt32", "Command"="", "Access"=enum."Read Only", "Range Table"="", "Read Callback"="", "Write Callback"="", "Range Callback"="", "Check Callback"="", "Rngtable Callback"="", "Coerce Callback"="", "Supported Models"="", "Instrument Options"="", "Check Status Callback"="", "Flags"=0, "Help"="Scheduled Slot Allocation."}, {"Level"=4, "Class Only"=FALSE, "Identifier"="RSCMWXPNRFR1M_ATTR_COMMON_PUSCH_ALLOCATION", "Descriptive Name"="Common PUSCH Allocation", "Data Type"=enum."RawString", "Command"="CONF:NRS:MEAS{instance}:CC{CC}:ALL{Allocation}:PUSC", "Access"=enum."Read/Write", "Range Table"="", "Read Callback"="", "Write Callback"="", "Range Callback"="", "Check Callback"="", "Rngtable Callback"="", "Coerce Callback"="", "Supported Models"="", "Instrument Options"="", "Check Status Callback"="", "Flags"=0, "Help"="Specifies settings related to the PUSCH allocation, for carrier <no>, allocation <a>.\n\nSyntax:\nCONFigure:NRSub:MEAS<i>[:CC<no>]:ALLocation<a>:PUSCh <MappingType>, <NoSymbols>, <StartSymbol>, <Auto>, <NoRBs>, <StartRB>, <ModScheme>\n\n<MappingType>\nPUSCH mapping type\nValid Values:\nA\nB\n  \n<NoSymbols>\nNumber of allocated OFDM symbols in each uplink slot.\nnumeric\nValid Values: 4 to 14 \n \n<StartSymbol>\nIndex of the first allocated symbol in each uplink slot.\nFor mapping type A, only 0 is allowed.\nnumeric\nValid Values: 0 to 10\n\n<Auto>\nAutomatic detection of <NoRBs> and <StartRB>\nValid Values: OFF | ON\n\n<NoRBs>\nNumber of allocated UL RBs.\nnumeric\nValid Values: 1 to 273 \n\n<StartRB>\nIndex of the first allocated RB.\nnumeric\nValid Values: 0 to 273\n\n<ModScheme>\nModulation scheme\nValid Values:\nAUTO - Auto\nBPSK - pi/2-BPSK\nBPWS - pi/2-BPSK with shaping\nQPSK - QPSK\nQ16 - 16-QAM\nQ64 - 64-QAM\nQ256 - 256-QAM\n\nAvailable Repeated Capabilities:\ninstance: i0, i1, i2, i3, i4, i5, i6, i7, i8, i9, i10, i11, i12, i13, i14, i15, i16, i17, i18, i19, i20, i21, i22, i23, i24, i25, i26, i27, i28, i29, i30, i31, i32\r\nCC: cc1, cc2\r\nAllocation: alloc1\r\n\nRemote-control command(s):\nCONFigure:NRSub:MEAS<i>[:CC<no>]:ALLocation<a>:PUSCh"}, {"Level"=4, "Class Only"=FALSE, "Identifier"="RSCMWXPNRFR1M_ATTR_ADDITIONAL_PUSCH_ALLOCATION", "Descriptive Name"="Additional PUSCH Allocation", "Data Type"=enum."ViInt32", "Command"="CONF:NRS:MEAS{instance}:CC{CC}:ALL{Allocation}:PUSC:ADD", "Access"=enum."Read/Write", "Range Table"="", "Read Callback"="", "Write Callback"="", "Range Callback"="", "Check Callback"="", "Rngtable Callback"="", "Coerce Callback"="", "Supported Models"="", "Instrument Options"="", "Check Status Callback"="", "Flags"=0, "Help"="Configures special PUSCH settings, for carrier <no>, allocation <a>.\n\nAvailable Repeated Capabilities:\ninstance: i0, i1, i2, i3, i4, i5, i6, i7, i8, i9, i10, i11, i12, i13, i14, i15, i16, i17, i18, i19, i20, i21, i22, i23, i24, i25, i26, i27, i28, i29, i30, i31, i32\r\nCC: cc1, cc2\r\nAllocation: alloc1\r\n\nRemote-control command(s):\nCONFigure:NRSub:MEAS<i>[:CC<no>]:ALLocation<a>:PUSCh:ADDitional"}, {"Level"=4, "Class Only"=FALSE, "Identifier"="RSCMWXPNRFR1M_ATTR_DR_MS_SEQUENCE_GENERATION", "Descriptive Name"="DR-MS Sequence Generation", "Data Type"=enum."RawString", "Command"="CONF:NRS:MEAS{instance}:CC{CC}:ALL{Allocation}:PUSC:SGEN", "Access"=enum."Read/Write", "Range Table"="", "Read Callback"="", "Write Callback"="", "Range Callback"="", "Check Callback"="", "Rngtable Callback"="", "Coerce Callback"="", "Supported Models"="", "Instrument Options"="", "Check Status Callback"="", "Flags"=0, "Help"="Configures the initialization of the DM-RS sequence generation, for carrier <no>, allocation <a>.\n\nSyntax:\nCONFigure:NRSub:MEAS<i>[:CC<no>]:ALLocation<a>:PUSCh:SGENeration <Initialization>, <DMRSID>, <N_SCID>\n\n<Initialization>\nUsed ID\nValid Values:\nPHY - cell ID used\nDID - DMRS ID used\n \n<DMRSID>\nID for <Initialization> = DMRSid.\nnumeric\nValid Values: 0 to 65535 \n\n<N_SCID>\nParameter nSCID.\nnumeric\nValid Values: 0 to 1\n\nAvailable Repeated Capabilities:\ninstance: i0, i1, i2, i3, i4, i5, i6, i7, i8, i9, i10, i11, i12, i13, i14, i15, i16, i17, i18, i19, i20, i21, i22, i23, i24, i25, i26, i27, i28, i29, i30, i31, i32\r\nCC: cc1, cc2\r\nAllocation: alloc1\r\n\nRemote-control command(s):\nCONFigure:NRSub:MEAS<i>[:CC<no>]:ALLocation<a>:PUSCh:SGENeration"}, {"Level"=3, "Class Only"=TRUE, "Identifier"="", "Descriptive Name"="Signaling", "Data Type"=enum."ViInt32", "Command"="", "Access"=enum."Read Only", "Range Table"="", "Read Callback"="", "Write Callback"="", "Range Callback"="", "Check Callback"="", "Rngtable Callback"="", "Coerce Callback"="", "Supported Models"="", "Instrument Options"="", "Check Status Callback"="", "Flags"=0, "Help"="Contains attributes for Signaling."}, {"Level"=4, "Class Only"=FALSE, "Identifier"="RSCMWXPNRFR1M_ATTR_SIGNALING_PHYSICAL_CELL_ID", "Descriptive Name"="Signaling Physical Cell ID", "Data Type"=enum."RawString", "Command"="SIGN:NRAD:CELL:PCID", "Access"=enum."Write Only", "Range Table"="", "Read Callback"="", "Write Callback"="", "Range Callback"="", "Check Callback"="", "Rngtable Callback"="", "Coerce Callback"="", "Supported Models"="", "Instrument Options"="", "Check Status Callback"="", "Flags"=0, "Help"="Defines the physical cell ID.\n\nSyntax:\n[CONFigure:]SIGNaling:NRADio:CELL:PCID <CellName>, <Id>\n\nAvailable Repeated Capabilities:\nNone\n\nRemote-control command(s):\n[CONFigure:]SIGNaling:NRADio:CELL:PCID"}, {"Level"=4, "Class Only"=FALSE, "Identifier"="RSCMWXPNRFR1M_ATTR_HIDDEN_QUERY_SIGNALING_PHYSICAL_CELL_ID", "Descriptive Name"="Query Signaling Physical Cell ID", "Data Type"=enum."ViInt32", "Command"="SIGN:NRAD:CELL:PCID?", "Access"=enum."Read Only", "Range Table"="", "Read Callback"="", "Write Callback"="", "Range Callback"="", "Check Callback"="", "Rngtable Callback"="", "Coerce Callback"="", "Supported Models"="", "Instrument Options"="", "Check Status Callback"="", "Flags"=8, "Help"="Queries the physical cell ID.\n\nSyntax:\n[CONFigure:]SIGNaling:NRADio:CELL:PCID? <CellName>\n\nParameters:\n<CellName>\nString\n\nAvailable Repeated Capabilities:\nNone\n\nRemote-control command(s):\n[CONFigure:]SIGNaling:NRADio:CELL:PCID?"}, {"Level"=4, "Class Only"=FALSE, "Identifier"="RSCMWXPNRFR1M_ATTR_SIGNALING_ADDITIONAL_SPECTRUM_EMISSION", "Descriptive Name"="Signaling Additional Spectrum Emission", "Data Type"=enum."RawString", "Command"="SIGN:NRAD:CELL:RFS:ASEM", "Access"=enum."Write Only", "Range Table"="", "Read Callback"="", "Write Callback"="", "Range Callback"="", "Check Callback"="", "Rngtable Callback"="", "Coerce Callback"="", "Supported Models"="", "Instrument Options"="", "Check Status Callback"="", "Flags"=0, "Help"="Sets the parameter 'AdditionalSpectrumEmission', signaled to the UE if the value is not OFF.\n\nSyntax:\n[CONFigure:]SIGNaling:NRADio:CELL:RFSettings:ASEMission <CellName>, <ASEmission>\n\nAvailable Repeated Capabilities:\nNone\n\nRemote-control command(s):\n[CONFigure:]SIGNaling:NRADio:CELL:RFSettings:ASEMission"}, {"Level"=4, "Class Only"=FALSE, "Identifier"="RSCMWXPNRFR1M_ATTR_HIDDEN_QUERY_SIGNALING_ADDITIONAL_SPECTRUM_EMISSION", "Descriptive Name"="Query Signaling Additional Spectrum Emission", "Data Type"=enum."ViInt32", "Command"="SIGN:NRAD:CELL:RFS:ASEM?", "Access"=enum."Read Only", "Range Table"="", "Read Callback"="", "Write Callback"="", "Range Callback"="", "Check Callback"="", "Rngtable Callback"="", "Coerce Callback"="", "Supported Models"="", "Instrument Options"="", "Check Status Callback"="", "Flags"=8, 
